vi "ZLIB Compress Files__ogtk.vi"(6 "password (none)":string, 7 "append (create new)":T1, 8 "error in (no error)":errorcluster, 9 "internal names (file name without path)":path[](array[path]), 10 "file names":path[](array[path]), 11 "archive name (file dialog)":path) -> (0 "error out":errorcluster, 3 "archive name out":path)   [LabVIEW 2018]
doc: "This function compresses a number of files into a ZIP file. Thearchive name must be defined and if no archive name is passed to the function it will prompt the user for such a archive name with the file dialog.\n\npassword, if not empty, will encrypt all the newly added files in the archive in such a way that they can only be extracted with the password later on."
uses:
  <userlib>/_OpenG.lib/file/file.llb/Strip Path - Arrays__ogtk.vi
  <userlib>/_OpenG.lib/lvzip/lvzip.llb/ZLIB Store File__ogtk.vi
  <userlib>/_OpenG.lib/file/file.llb/Valid Path - Traditional__ogtk.vi
  <userlib>/_OpenG.lib/lvzip/lvzip.llb/ZLIB Open ZIP Mode__ogtk.ctl
panel:
  # "Please visit http://www.OpenG.org to learn about the\nOpen Source LabVIEW software movement.\n\nNOTICE -- YOU MUST LEAVE THIS NOTICE IN PLACE.  PER THE TERMS OF THE LICENSE BELOW, YOU MAY SUBLICENSE THIS SOFTWARE \nIN ANY WAY THAT DOES NOT CONFLICT WITH THIS LICENSE.\n\n### BSD License (http://www.opensource.org/licenses/bsd-license.php) Begin ###\n \nCopyright (C) 2002-2004 Rolf Kalbermatter rolf.kalbermatter@citeng.com\nCopyright (C) 2002 Jim Kring jim@jimkring.com\n\nAll rights reserved.\n\nRedistribution and use in source and binary forms, with or without modification, are permitted provided that the following conditions are met:\n\n    * Redistributions of source code must retain the above copyright notice, this list of conditions and the following disclaimer.\n    * Redistributions in binary form must reproduce the above copyright notice, this list of conditions and the following disclaimer in the \n       documentation and/or other materials provided with the distribution.\n    * Neither the name of SciWare, James Kring, Inc., nor the names of its contributors may be used to endorse or promote products derived \n       from this software without specific prior written permission.\n\nTHIS SOFTWARE IS PROVIDED BY THE COPYRIGHT HOLDERS AND CONTRIBUTORS \"AS IS\" AND ANY EXPRESS OR IMPLIED WARRANTIES, \nINCLUDING, BUT NOT LIMITED TO, THE IMPLIED WARRANTIES OF MERCHANTABILITY AND FITNESS FOR A PARTICULAR PURPOSE ARE \nDISCLAIMED. IN NO EVENT SHALL THE COPYRIGHT OWNER OR CONTRIBUTORS BE LIABLE FOR ANY DIRECT, INDIRECT, INCIDENTAL,\n SPECIAL, EXEMPLARY, OR CONSEQUENTIAL DAMAGES (INCLUDING, BUT NOT LIMITED TO, PROCUREMENT OF SUBSTITUTE GOODS OR \nSERVICES; LOSS OF USE, DATA, OR PROFITS; OR BUSINESS INTERRUPTION) HOWEVER CAUSED AND ON ANY THEORY OF LIABILITY, \nWHETHER IN CONTRACT, STRICT LIABILITY, OR TORT (INCLUDING NEGLIGENCE OR OTHERWISE) ARISING IN ANY WAY OUT OF THE USE \nOF THIS SOFTWARE, EVEN IF ADVISED OF THE POSSIBILITY OF SUCH DAMAGE.\n\n### BSD License End ###"
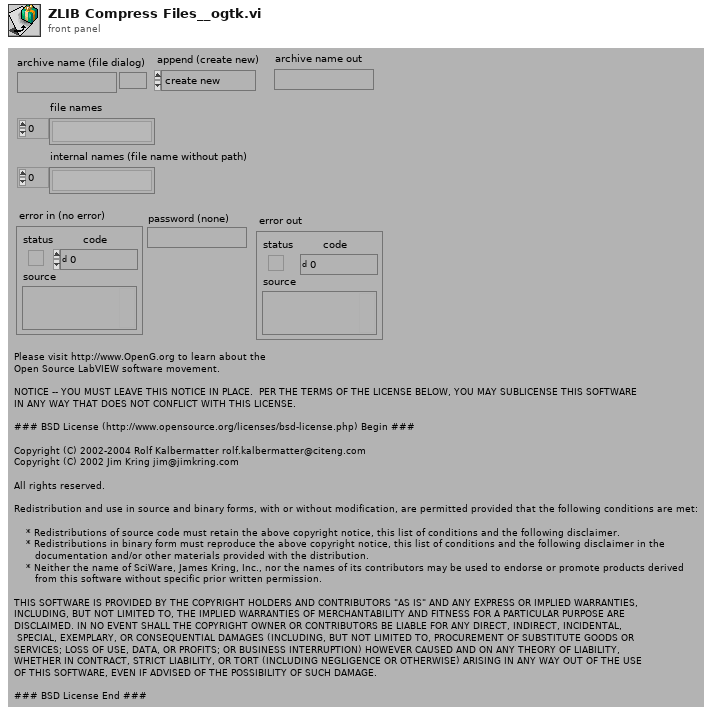
[diagram p1: front panel]
types:
  T1 = typedef "ZLIB Open ZIP Mode__ogtk.ctl" = enum16{"create new", "append to end", "append to archive"}
  T2 = enum32{"existing file", "new file", "new or existing file", "existing dir", "new dir", "new or existing dir", "existing file (use LLBs)", "new file (use LLBs)", "new or existing file (use LLBs)", "new or existing file or directory (use LLBs)", "existing dir (use LLBs)", "new dir (use LLBs)", "new or existing dir (use LLBs)", "existing file or dir", "new file or dir", "new or existing file or dir", "existing file or dir (use LLBs)", "new file or dir (use LLBs)"}
  T3 = typedef "ZLIB Zip Handle__ogtk.ctl" = refnum<k1>
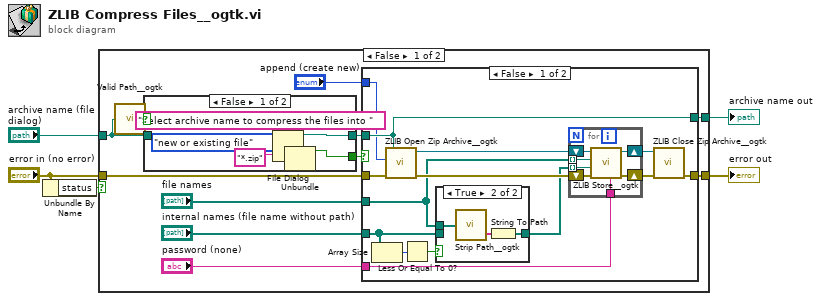
[diagram p0: block diagram]
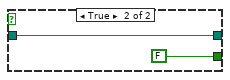
[diagram p2: hidden frame]
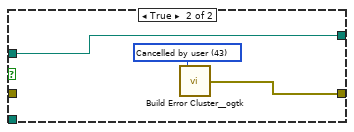
[diagram p4: hidden frame]
diagram:
  n1 = Unbundle By Name("error in (no error)") -> ("status"=w4:bool)
  n2 = case shown="False" w4 {
    tunnel: "archive name (file dialog)" -> [w13 w52]
    tunnel: "error in (no error)" -> [w11 w53]
    tunnel: [w12 w53] -> w2
    tunnel: [w10 w52] -> w1
    frame False {
      n3 = call-poly <userlib>:"Valid Path__ogtk.vi"("path"=w13) -> ("valid"=w14:bool)
      n4 = case shown="False" w14 {
        tunnel: [w20 w23] -> w16
        tunnel: [w19 FALSE ("cancelled")] -> w15
        tunnel: w13 -> [_ w23]
        frame False {
          (unwired) T2."new or existing file" ("select mode (2)")
          n5 = File Dialog(6:"*.zip" ("default name"), 7:"Select archive name to compress the files into " ("prompt")) -> (0:w17:errorcluster, 1:w19:bool, 3:w20:path)  [unwired: 5 in, 1 out]
          n6 = Unbundle(w17) -> ()  [unwired: 3 out]
        }
        frame True {
        }
      }
      n7 = case shown="False" w15 {
        tunnel: w16 -> [w31 w49]
        tunnel: [w33 w51] -> w12
        tunnel: w11 -> [w32 _]
        tunnel: [w31 w49] -> w10
        tunnel: "file names" -> [w30 _]
        tunnel: "append (create new)" -> [w28 _]
        tunnel: "internal names (file name without path)" -> [w26 _]
        tunnel: "password (none)" -> [w24 _]
        frame False {
          n8 = Array Size(array=w26) -> (size(s)=w25:i32)
          n9 = call <userlib>:"ZLIB Open Zip Archive__ogtk.vi"("error in (no error)"=w32, "append (create new)"=w28, "archive name"=w31) -> ("error out"=w37:errorcluster, "zip Refnum"=w36:T3)  [unwired: 2 in, 1 out]
          n10 = Less Or Equal To 0?(x=w25) -> (x <= 0?=w27:bool)
          n11 = case shown="True" w27 {
            tunnel: w30 -> [_ w39]
            tunnel: [w38 w40] -> w29
            tunnel: w26 -> [w38 _]
            frame False {
            }
            frame True {
              n12 = call-poly <userlib>:"Strip Path__ogtk.vi"("path"=w39) -> ("name"=w41:string[])  [unwired: 1 out]
              n13 = String To Path(string=w41) -> (path=w40:path[])
            }
          }
          n14 = for {
            shift-right: [w46] -> w35
            shift-left: w36 -> [w48]
            shift-right: [w45] -> w34
            shift-left: w37 -> [w47]
            tunnel: w30 -> [w44] mode=indexing
            tunnel: w29 -> [w43] mode=indexing
            tunnel: w24 -> [w42]
            n15 = call-poly <userlib>:"ZLIB Store__ogtk.vi"("password (none)"=w42, "error in (no error)"=w47, "internal name (same as source name)"=w43, "source path"=w44, "zip Refnum"=w48) -> ("error out"=w45:errorcluster, "zip Refnum out"=w46:T3)  [unwired: 5 in]
          }
          n16 = call <userlib>:"ZLIB Close Zip Archive__ogtk.vi"("error in (no error)"=w34, "zip Refnum"=w35) -> ("error out"=w33:errorcluster)  [unwired: 4 in, 1 out]
        }
        frame True {
          w50 = 43 items=["No error", "Argument error", "Memory is full", "Out of zone", "End of file", "File already open", "Generic file I/O error", "File not found", "File permission error", "Disk is full", "Duplicate path", "Too many files open", "System feature not enabled", "Resource file not found", "Cannot add resource", "Resource not found", "Image not found", "Image memory error", "Pen does not exist", "Config type invalid", "Config token not found", "Config parse error", "Config memory error", "Bad external code format", "Bad external code offset", "External code not present", "Null window", "Destroy window error", "Null menu", "Print aborted", "Bad print record", "Print driver error", "Windows error during printing", "Memory error during printing", "Print dialog error", "Generic print error", "Invalid device refnum", "Device not found", "Device parameter error", "Device unit error", "Cannot open device", "Device call aborted", "Generic error", "Cancelled by user", "Object ID too low", "Object ID too high", "Object not in heap", "Unknown heap", "Unknown object (invalid DefProc)", "Unknown object (DefProc not in table)", "Message out of range", "Invalid (null) method", "Unknown message", "Manager call not supported", "Bad address", "Network operation in progress", "Network operation timed out", "Connection is busy", "Network attribute not supported", "Network error", "Address in use", "System out of memory", "Connection aborted", "Connection refused", "Not connected", "Already connected", "Connection closed", "Initialization error (interapplication manager)", "Bad occurrence", "Wait on unbound occurrence handler", "Occurrence queue overflow", "Datalog type conflict", "Unused", "Unrecognized type (interapplication manager)", "Memory corrupt", "Failed to make temporary DLL", "Old CIN version", "Drag socket not found", "Failed to load drop-object", "Failed to register OLE object", "Failed to release OLE object", "Format specifier type mismatch", "Unknown format specifier", "Too few format specifiers", "Too many format specifiers", "Scan failed", "Newer CIN version", "Error converting to variant", "Runtime menu error", "Password tampered", "Variant attribute not found", "Incompatible variant data type", "Event data is not available", "Event Store is not present", "Occurrence is not found", "Event Queue is not created", "Event info is not available", "Refnum passed is NULL", "Error retrieving Class GUID", "Error retrieving CoClass GUID", "Error retrieving TypeLib GUID.", "Bad built application magic bytes.", "Specific driver is different from the specific driver associated with the Logical Name.", "There is no session opened to the class driver.", "Max Error", "MAX - Error with config objects", "MAX - Error loading configuration", "MAX - Group not supported"]
          n17 = call <userlib>:"Build Error Cluster__ogtk.vi"("code"=w50) -> ("error out"=w51:errorcluster)  [unwired: 1 in]
        }
      }
    }
    frame True {
    }
  }
  "error out" <- w2
  "archive name out" <- w1
